vi "Variables.vi"(8 "error in (no error)":errorcluster, 10 "Value":variant, 11 "Command":T1(ring)) -> (0 "error out":errorcluster, 2 "Step Counter":i32, 3 "Out Message":string)   [LabVIEW 2017]
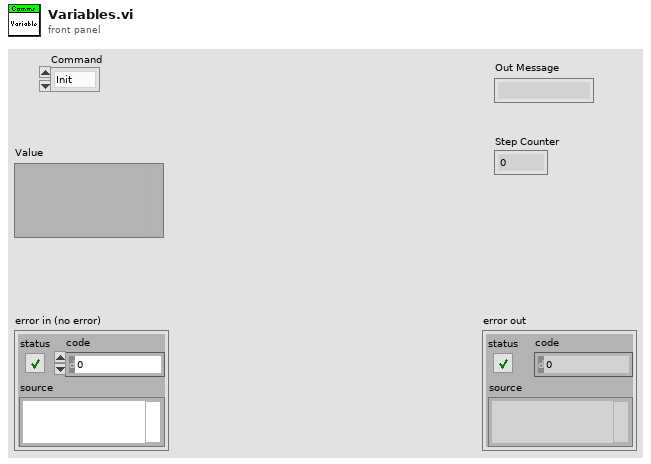
[diagram p1: front panel]
types:
  T1 = enum16{"Init", "Get", "Set Step Counter", "Insert Command", "Insert Now Command"}
  T2 = cluster{"Message Array":string[], "Num Messages":i32, "Step Counter":i32, "Added Commands":string[]}
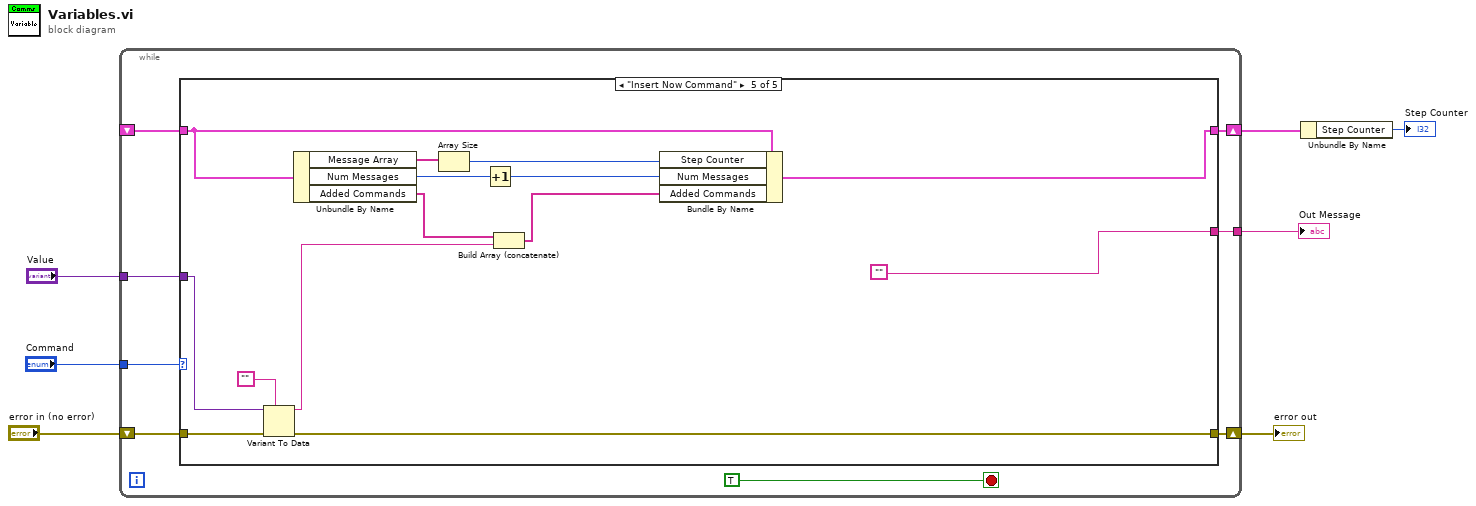
[diagram p0: block diagram]
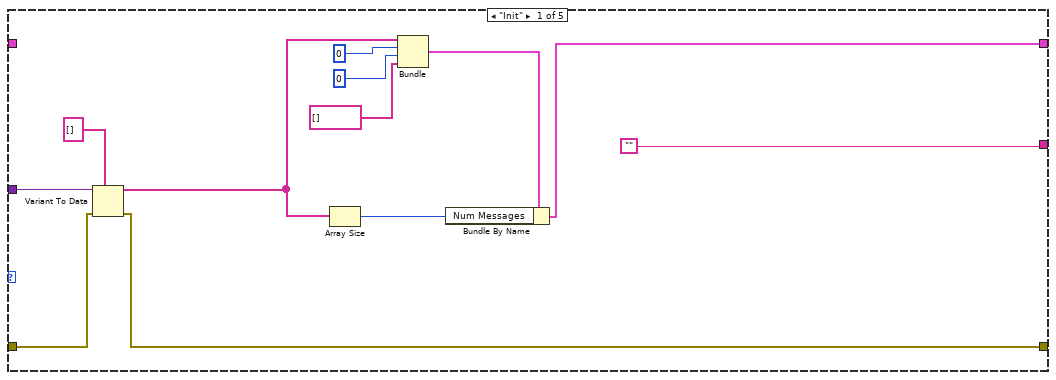
[diagram p2: hidden frame]
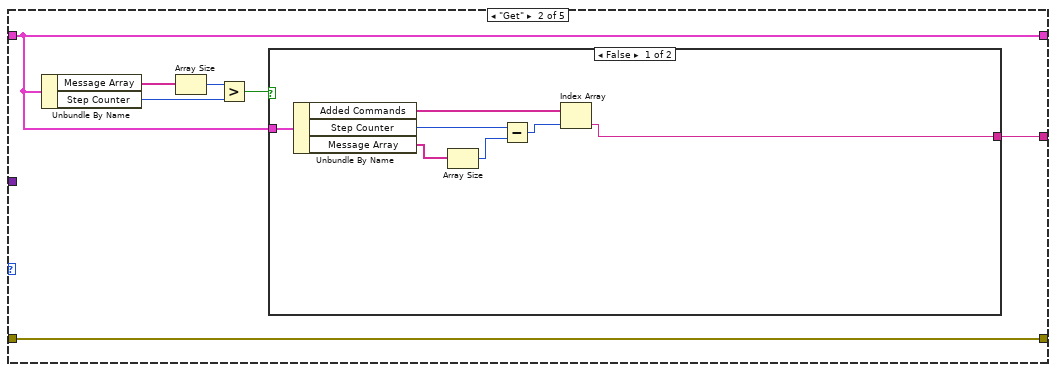
[diagram p3: hidden frame]
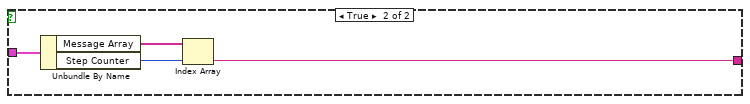
[diagram p4: hidden frame]
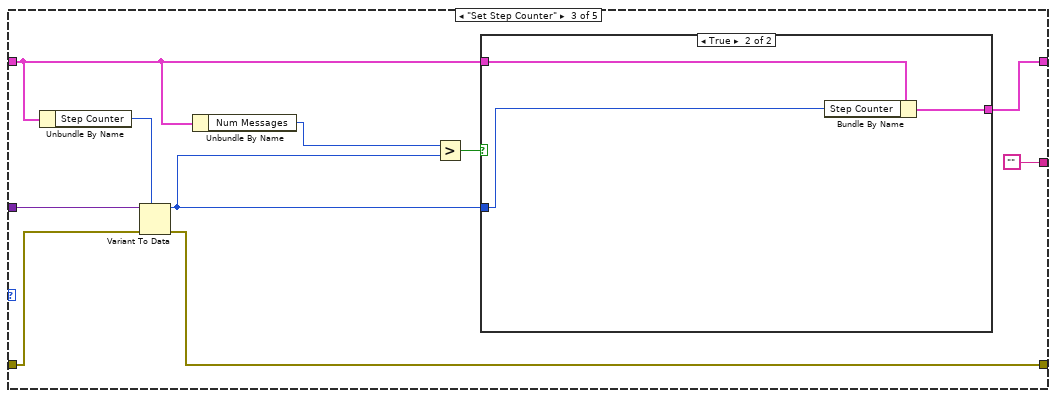
[diagram p5: hidden frame]
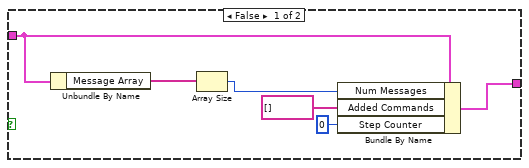
[diagram p6: hidden frame]
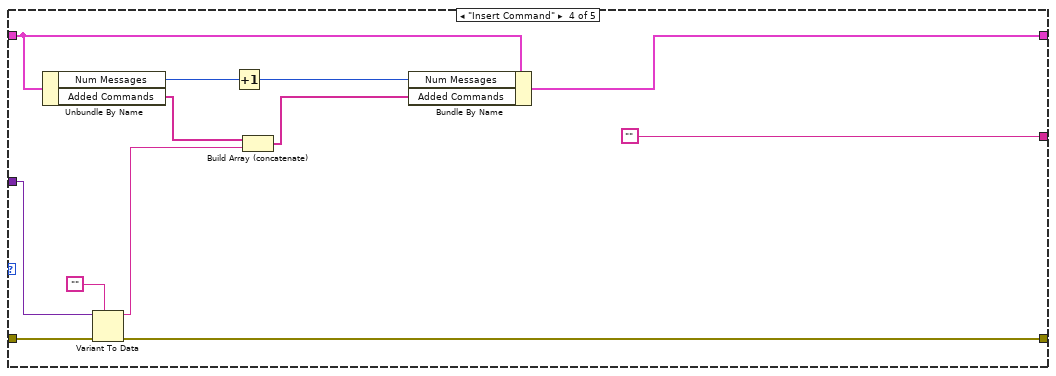
[diagram p7: hidden frame]
diagram:
  n1 = while {
    shift-right: [w14] -> w6
    shift-left: "error in (no error)" -> [w13]
    tunnel: "Command" -> [w8]
    shift-right: [w12] -> w2
    shift-left: _ -> [w11]
    tunnel: "Value" -> [w10]
    tunnel: [w9] -> w3
    stop <- TRUE stop-if-true
    n2 = case shown="\"Insert Now Command\"" w8 {
      tunnel: [w18 w28 w52 w66 w87] -> w14
      tunnel: w13 -> [w19 w28 w54 w72 w90]
      tunnel: [w25 w29 w48 w73 w82] -> w12
      tunnel: w11 -> [_ w29 w47 w76 w80]
      tunnel: w10 -> [w22 _ w55 w71 w89]
      tunnel: ["" w30 "" "" ""] -> w9
      frame "Init" {
        n3 = Variant To Data(error in=w19, type=string[] [] ("Message Array"), Variant=w22) -> (data=w20:string[], error out=w18:errorcluster)
        n4 = Array Size(array=w20) -> (size(s)=w24:i32)
        n5 = Bundle("Message Array"=w20, "Num Messages"=0, "Step Counter"=0, "Added Commands"=string[] []) -> (w26:T2)  [unwired: 1 in]
        n6 = Bundle By Name(cluster=w26, "Num Messages"=w24) -> (w25:T2)
      }
      frame "Get" {
        n7 = Unbundle By Name(w29) -> ("Message Array"=w34:string[], "Step Counter"=w32:i32)
        n8 = Array Size(array=w34) -> (size(s)=w33:i32)
        n9 = Greater?(x=w33, y=w32) -> (0:w31:bool)
        n10 = case shown="False" w31 {
          tunnel: [w35 w42] -> w30
          tunnel: w29 -> [w41 w45]
          frame False {
            n11 = Unbundle By Name(w41) -> ("Added Commands"=w37:string[], "Step Counter"=w39:i32, "Message Array"=w40:string[])
            n12 = Array Size(array=w40) -> (size(s)=w38:i32)
            n13 = Subtract(x=w39, y=w38) -> (x-y=w36:i32)
            n14 = Index Array(array=w37, index=w36) -> (element=w35:string)
          }
          frame True {
            n15 = Unbundle By Name(w45) -> ("Message Array"=w44:string[], "Step Counter"=w43:i32)
            n16 = Index Array(array=w44, index=w43) -> (element=w42:string)
          }
        }
      }
      frame "Set Step Counter" {
        n17 = Unbundle By Name(w47) -> ("Step Counter"=w53:i32)
        n18 = Variant To Data(error in=w54, type=w53, Variant=w55) -> (data=w49:i32, error out=w52:errorcluster)
        n19 = Unbundle By Name(w47) -> ("Num Messages"=w46:i32)
        n20 = Greater?(x=w46, y=w49) -> (0:w50:bool)
        n21 = case shown="True" w50 {
          tunnel: w47 -> [w58 w64]
          tunnel: w49 -> [_ w62]
          tunnel: [w61 w63] -> w48
          frame False {
            n22 = Unbundle By Name(w58) -> ("Message Array"=w57:string[])
            n23 = Array Size(array=w57) -> (size(s)=w56:i32)
            n24 = Bundle By Name(cluster=w58, "Num Messages"=w56, "Added Commands"=string[] [], "Step Counter"=0) -> (w61:T2)
          }
          frame True {
            n25 = Bundle By Name(cluster=w64, "Step Counter"=w62) -> (w63:T2)
          }
        }
      }
      frame "Insert Command" {
        n26 = Unbundle By Name(w76) -> ("Num Messages"=w75:i32, "Added Commands"=w69:string[])
        n27 = Variant To Data(error in=w72, type="", Variant=w71) -> (data=w68:string, error out=w66:errorcluster)
        n28 = Increment(x=w75) -> (x+1=w74:i32)
        n29 = Build Array (concatenate)(w69, w68) -> (w67:string[])
        n30 = Bundle By Name(cluster=w76, "Num Messages"=w74, "Added Commands"=w67) -> (w73:T2)
      }
      frame "Insert Now Command" {
        n31 = Variant To Data(error in=w90, type="", Variant=w89) -> (data=w81:string, error out=w87:errorcluster)
        n32 = Unbundle By Name(w80) -> ("Message Array"=w78:string[], "Num Messages"=w86:i32, "Added Commands"=w84:string[])
        n33 = Array Size(array=w78) -> (size(s)=w77:i32)
        n34 = Increment(x=w86) -> (x+1=w85:i32)
        n35 = Build Array (concatenate)(w84, w81) -> (w83:string[])
        n36 = Bundle By Name(cluster=w80, "Step Counter"=w77, "Num Messages"=w85, "Added Commands"=w83) -> (w82:T2)
      }
    }
  }
  "error out" <- w6
  "Out Message" <- w3
  n37 = Unbundle By Name(w2) -> ("Step Counter"=→"Step Counter":i32)
